vi "NI6008 TestCtrl Ctrl.vi"(8 "error in (no error)":errorcluster, 10 "On/Off":bool, 11 "Actor_NI6008 in":refnum<class "Actor_NI6008.lvclass">) -> (0 "error out":errorcluster, 3 "Actor_NI6008 out":refnum<class "Actor_NI6008.lvclass">)   [LabVIEW 2020, in "Actor_NI6008.lvlib" / "Actor_NI6008.lvclass"]
uses:
  Actor_NI6008.lvclass
  C:/Program Files/National Instruments/LabVIEW 2020/vi.lib/ActorFramework/Actor/Actor.lvclass
  <vilib>/ActorFramework/Actor/Actor.lvclass/Actor.ctl
  Actor_NI6008.lvclass/Actor_NI6008.ctl
  I_NI6008 Messages/NI6008 Status Report Msg/NI6008 Status Report Msg.lvclass/NI6008 Status Report Msg.ctl
  <vilib>/ActorFramework/Message Enqueuer/Message Enqueuer.lvclass/Message Enqueuer.ctl
  <vilib>/DAQmx/write.llb/DAQmx Write (Digital Bool 1Line 1Point).vi
  <vilib>/ActorFramework/Message Enqueuer/Enqueue.vi
  I_NI6008 Messages/NI6008 Status Report Msg/NI6008 Status Report Msg.lvclass
  C:/Program Files/National Instruments/LabVIEW 2020/vi.lib/ActorFramework/Message/Message.lvclass
  <vilib>/DAQmx/miscellaneous.llb/DAQmx Fill In Error Info.vi
  <vilib>/ActorFramework/Message Priority Queue/Priority Enqueue.vi
  <vilib>/ActorFramework/Actor/Actor.lvclass
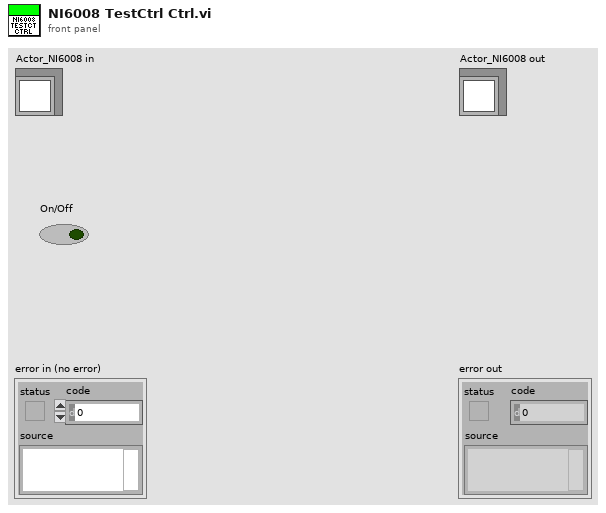
[diagram p1: front panel]
types:
  T1 = cluster{"Msg":string, "DO":bool[], "AI":dbl, "NI6008 Error":errorcluster}
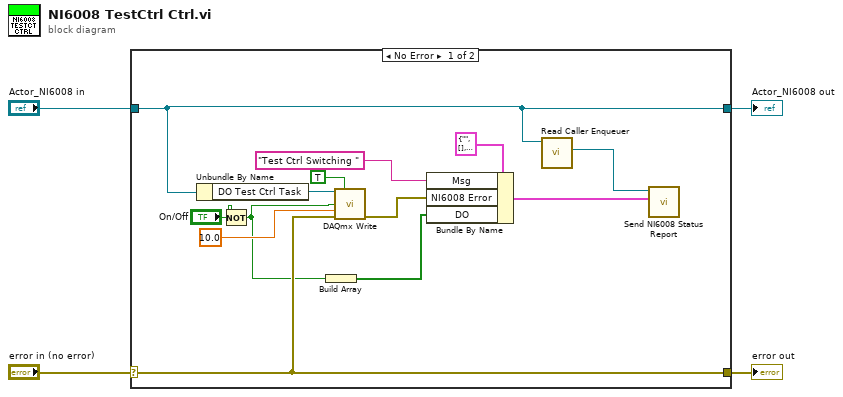
[diagram p0: block diagram]
diagram:
  n1 = case shown="No Error" "error in (no error)" {
    selector: "error in (no error)" -> [w7 w19]
    tunnel: [w7 w19] -> w3
    tunnel: [w8 w18] -> w1
    tunnel: "Actor_NI6008 in" -> [w8 w18]
    frame No Error {
      n2 = Unbundle By Name(w8) -> ("DO Test Ctrl Task"=w13:refnum<k21>)
      n3 = Not(x="On/Off") -> (.not. x?=w5:bool)
      n4 = Build Array(w5) -> (w10:bool[])
      n5 = call-poly <vilib>:"DAQmx Write.vi"("task/channels in"=w13, "auto start"=TRUE, "data"=w5, "timeout"=10.0, "error in"=w7) -> ("error out"=w9:errorcluster)  [unwired: 8 in, 2 out]
      n6 = Bundle By Name(cluster=T1 {"Msg"="", "DO"=[], "AI"=0.0, "NI6008 Error"={"status"=FALSE, "code"=0, "source"=""}} ("Data"), "Msg"="Test Ctrl Switching ", "NI6008 Error"=w9, "DO"=w10) -> (w15:T1)
      n7 = call <vilib>:"Read Caller Enqueuer.vi"("Actor"=w8) -> ("Caller Enqueuer"=w14:refnum<class "Message Enqueuer.lvclass">)  [unwired: 10 in]
      n8 = call "Send NI6008 Status Report.vi"("Data"=w15, "Message Enqueuer"=w14) -> ()  [unwired: 8 in, 2 out]
    }
    frame Error {
    }
  }
  "error out" <- w3
  "Actor_NI6008 out" <- w1
